vi "2019-05-09_shift_register.vi"() -> ()   [LabVIEW 2018]
panel:
  out "Data 2":i32
  out "Data 1":i32
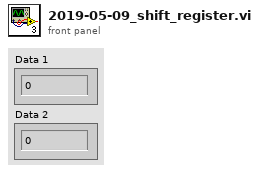
[diagram p1: front panel]
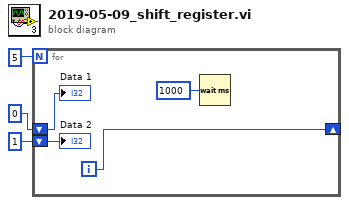
[diagram p0: block diagram]
diagram:
  n1 = for {
    N: 5 -> [_]
    shift-right: [w5] -> _
    shift-left: 0 -> [w7]
    shift-left: 1 -> [w6]
    i -> [w5]
    n2 = Wait (ms)(milliseconds to wait=u32 1000 ("대기 시간 (ms)")) -> ()  [unwired: 1 out]
    "Data 1" <- w7
    "Data 2" <- w6
  }
